vi "testrandled.vi"() -> ()   [LabVIEW 2012]
uses:
  <vilib>/Platform/TimedLoop/XDataNode/XDataNode.xnode
  <vilib>/Platform/TimedLoop/XDataNode/nitl_modes.ctl
  <vilib>/Platform/TimedLoop/XDataNode/XDNodeRunTimeDep.lvlib
  <vilib>/Platform/TimedLoop/XDataNode/wakeup.ctl
  <vilib>/Platform/TimedLoop/XDataNode/timing_clust.ctl
  <vilib>/eio/EIONode/EIONode.xnode
  <vilib>/rvi/eio/common/nirviEmuTemplateMethod_errors.vi
panel:
  out "Wait counter":u32
  out "Is Test Pulse?":bool
  out "Total number of pulses sent":u64
  in  "Testpulse Time Delay (20 ns ticks)":u32=15
  in  "Testpulse duration (20 ns ticks)":u32=1
  in  "Testpulser On/Off":bool
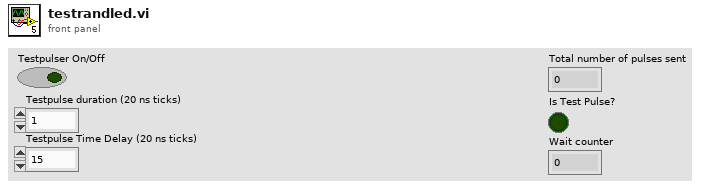
[diagram p1: front panel]
types:
  T1 = typedef "XDNodeRunTimeDep.lvlib/timing_clust.ctl" = cluster{"Expected End [f-1]":u64, "Actual End [f-1]":u64, "Finished Late? [f-1]":bool, "Expected End [i-1]":u64, "Actual End [i-1]":u64, "Finished Late? [i-1]":bool, "Expected Start [i]":u64, "Actual Start [i]":u64, "Expected Start [f]":u64, "Actual Start [f]":u64, "Source Name":string, "Structure Name":string, "Period":i64, "Deadline":i64, "Offset":i64, "Start":i64, "Priority":i32, "Timeout":i32, "Mode":T2, "Wakeup Reason":T3, "Error":errorcluster, "Source Type":string, "Secondary Source Type":string, "Global End Time":u64, "Global Start Time":u64, "Frame Duration":u64, "Iteration Duration":u64, "Assigned CPU":i32, "I/O Scan Engine Mode":u32}
  T2 = typedef "XDNodeRunTimeDep.lvlib/nitl_modes.ctl" = enum32{"No Change", "Process missed periods, maintain original phase", "Discard missed periods, maintain original phase", "Process missed periods, ignore original phase", "Discard missed periods, ignore original phase"}
  T3 = typedef "XDNodeRunTimeDep.lvlib/wakeup.ctl" = enum32{"Normal", "Aborted", "Asynchronous wakeup", "Timing source error", "Timed loop error", "Timeout"}
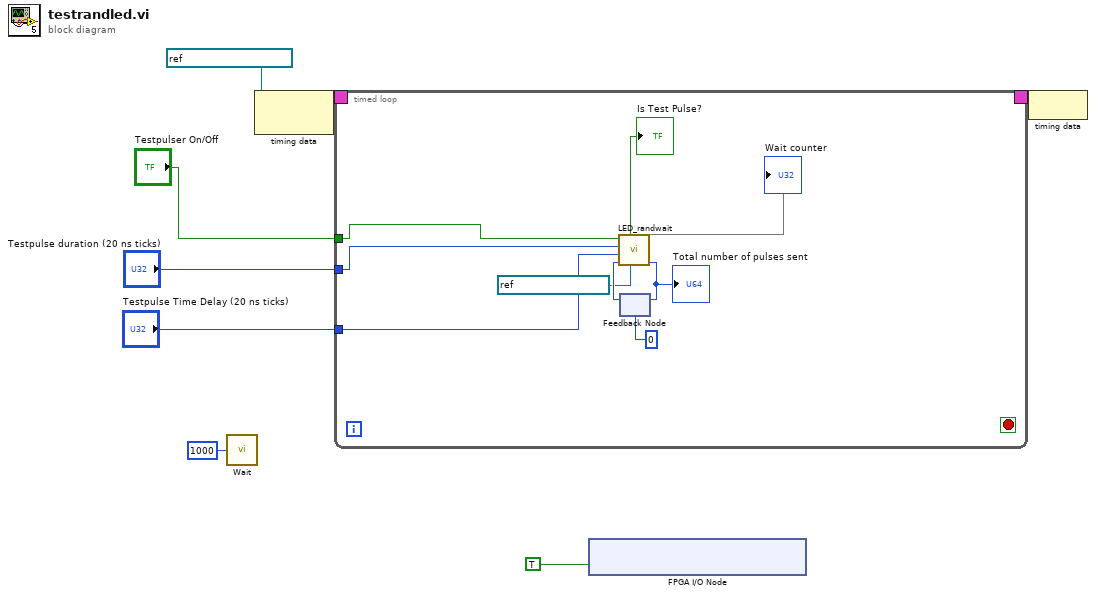
[diagram p0: block diagram]
diagram:
  n1 = call "Wait"("Count(mSec)"=u32 1000) -> ()  [unwired: 1 out]
  n2 = node-c288(refnum<k21> "IO Module Clock 0" ("Source Name")) -> (w6:T1)
  n3 = timed-loop {
    tunnel: "Testpulser On/Off" -> [w9]
    tunnel: "Testpulse duration (20 ns ticks)" -> [w17]
    tunnel: "Testpulse Time Delay (20 ns ticks)" -> [w16]
    timing: w6 -> [_]
    timing-out: [_] -> w5
    stop <- _ stop-if-true
    n4 = feedback #1(u64 0 ("Total number of pulses sent")) -> (w14:u64)
    n5 = call "LED_randwait.vi"("FPGA I/O In"=refnum<k21> "IO Module\\D0 0", "seed"=w14, "Testpulse Time Delay (20 ns ticks)"=w16, "Testpulse duration (20 ns ticks)"=w17, "Testpulser On/Off"=w9) -> ("Total number of pulses sent"=w15:u64, 5:→"Wait counter", "Is Test Pulse?"=→"Is Test Pulse?":bool)  [unwired: 4 in]
    "Total number of pulses sent" <- w15
    n6 = feedback-in #1(w15) -> ()
  }
  n7 = xnode "FPGA I/O Node"("IO Module\\Digital Output Enable"=TRUE ("Testpulser On/Off")) -> ()  [unwired: 1 in, 1 out]
  n8 = node-c288(w5) -> ()
